vi "WSVCAP SHL Host LL Get Read Byte Parameter.vi"(11 "error in (no error)":errorcluster, 14 "FPGA":T1) -> (4 "Read Data In":u64, 15 "error out":errorcluster)   [LabVIEW 2012]
uses:
  Type Defs/WSVCAP SHL I2C FPGA Enum.ctl
  Type Defs/WSVCAP SHL Top Level Control Operation Enum.ctl
  Type Defs/WSVCAP SHL Top Level Control Enum.ctl
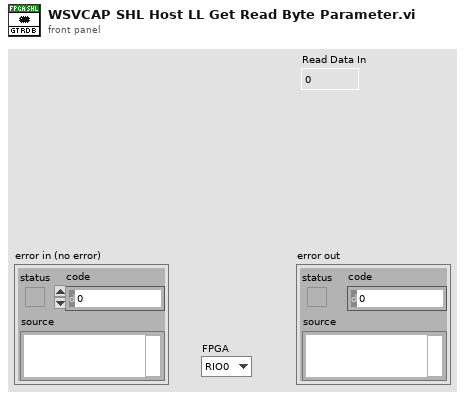
[diagram p1: front panel]
types:
  T1 = typedef "WSVCAP SHL I2C FPGA Enum.ctl" = enum16{"RIO0", "RIO1"}
  T2 = typedef "WSVCAP SHL Top Level Control Enum.ctl" = enum16{"Start", "Cmd", "Transaction", "Wait Ticks", "Socket Mask", "UUT Set", "Slave Address", "Sub Address", "Bytes to Write", "Bytes to Read", "Write Data", "Write Flag", "Read Data", "Read Flag", "Ack Read", "Read Status Flag", "Ack Read Status", "Status", "Cycle Count", "Stop Cycle", "Exit"}
  T3 = typedef "WSVCAP SHL Top Level Control Operation Enum.ctl" = enum16{"Initialize", "Set Control", "Read Control", "Close"}
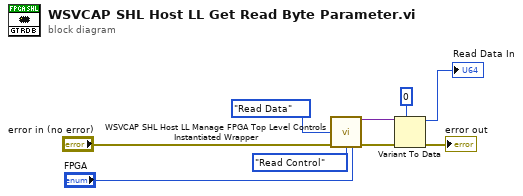
[diagram p0: block diagram]
diagram:
  n1 = call "WSVCAP SHL Host LL Manage FPGA Top Level Controls Instantiated Wrapper.vi"("FPGA Top Level Control"=WSVCAP_SHL_Top_Level_Control_Enum."Read Data", "error in (no error)"="error in (no error)", "Operation"=WSVCAP_SHL_Top_Level_Control_Operation_Enum."Read Control", "FPGA"="FPGA") -> ("Value Out"=w4:variant, "error out"=w6:errorcluster)  [unwired: 10 in]
  n2 = Variant To Data(error in=w6, type=u64 0 ("Read Data In"), Variant=w4) -> (data=→"Read Data In":u64, error out=→"error out":errorcluster)
